vi "File List Get first file.vi"(11 "File List in":refnum<class "File List.lvclass">) -> (1 "Current file index out":i32, 2 "Current file out":path, 3 "File List out":refnum<class "File List.lvclass">)   [LabVIEW 2011, in "COSYLib.lvlib" / "File List.lvclass"]
doc: "Activates and returns the first file.\nIf there are no files in the list, an empty path and the index \"-1\" are returned."
uses:
  File List.lvclass
  File List.lvclass/File List.ctl
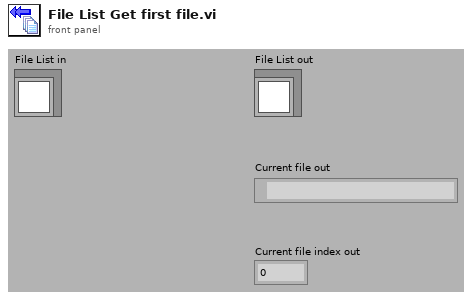
[diagram p1: front panel]
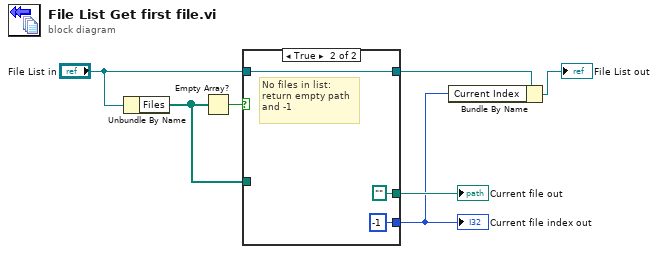
[diagram p0: block diagram]
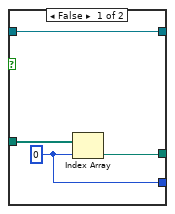
[diagram p2: hidden frame]
diagram:
  n1 = Unbundle By Name("File List in") -> ("Files"=w4:path[])
  n2 = Empty Array?(array=w4) -> (empty?=w5:bool)
  n3 = case shown="True" w5 {
    tunnel: "File List in" -> [w8 w13]
    tunnel: [w8 w13] -> w3
    tunnel: [w10 path ""] -> w6
    tunnel: w4 -> [w11 _]
    tunnel: [w9 -1] -> w1
    frame False {
      w9 = 0
      n4 = Index Array(array=w11, index=w9) -> (element=w10:path)
    }
    frame True {
      # "No files in list:\nreturn empty path\nand -1"
    }
  }
  "Current file out" <- w6
  "Current file index out" <- w1
  n5 = Bundle By Name(cluster=w3, "Current Index"=w1) -> (→"File List out":refnum<class "File List.lvclass">)
